vi "Individual Cartesian Measurements.vi"(6 "Forces In":dbl[](array[numeric]), 7 "LBCB Number":T1, 8 "error in (no error)":errorcluster, 9 "Displacements In":dbl[](array[numeric]), 11 "DAO Actions":T2) -> (0 "error out":errorcluster, 1 "Displacements Out":dbl[](array[numeric]), 5 "Forces Out":dbl[](array[numeric]))   [LabVIEW 2009]
uses:
  Data Access Objects/Metadata/DAO Actions.ctl
  Data Access Objects/Metadata/LBCB Number.ctl
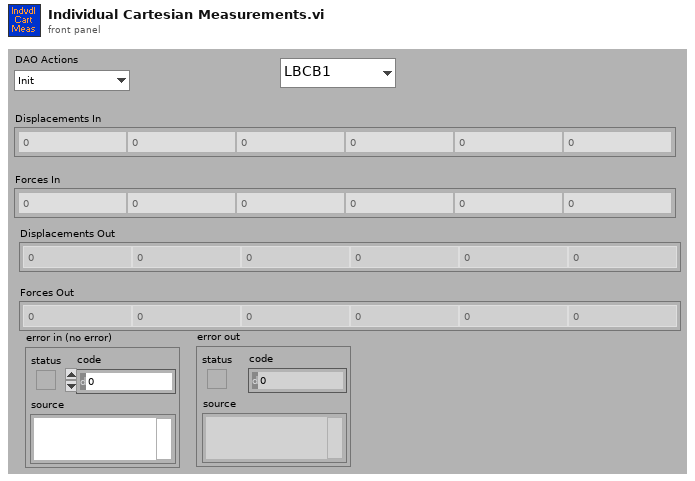
[diagram p1: front panel]
types:
  T1 = typedef "LBCB Number.ctl" = enum16{"LBCB1", "LBCB2"}
  T2 = typedef "DAO Actions.ctl" = enum16{"Init", "Get", "Set"}
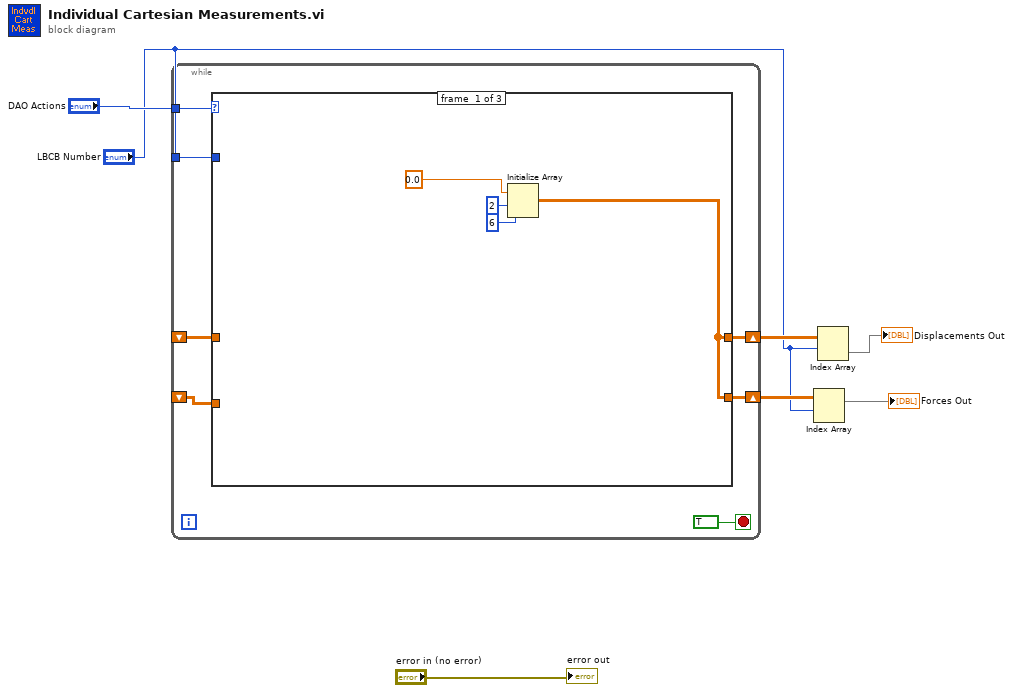
[diagram p0: block diagram]
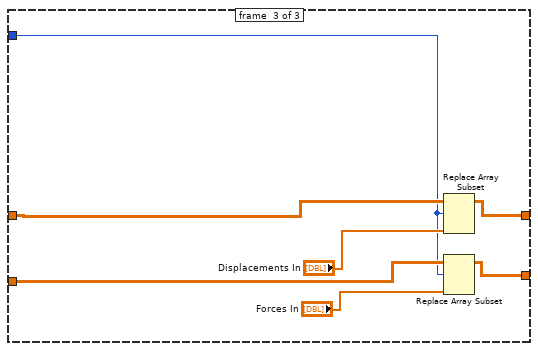
[diagram p3: hidden frame]
diagram:
  n1 = while {
    tunnel: "DAO Actions" -> [w13]
    shift-right: [w12] -> w5
    shift-left: _ -> [w11]
    tunnel: "LBCB Number" -> [w10]
    shift-right: [w9] -> w3
    shift-left: _ -> [w8]
    stop <- TRUE stop-if-true
    n2 = case shown="\"Get\"" w13 {
      tunnel: [w15 w20 w26] -> w12
      tunnel: w11 -> [_ w20 w27]
      tunnel: w10 -> [_ _ w21]
      tunnel: [w15 w19 w22] -> w9
      tunnel: w8 -> [_ w19 w23]
      frame #0 {
        n3 = Initialize Array(0.0, 2 ("dimension size"), 6 ("dimension size")) -> (w15:dbl[][])
      }
      frame #1 {
      }
      frame #2 {
        n4 = Replace Array Subset(array=w27, new element="Displacements In", index (row)=w21) -> (w26:dbl[][])  [unwired: 1 in]
        n5 = Replace Array Subset(array=w23, new element="Forces In", index (row)=w21) -> (w22:dbl[][])  [unwired: 1 in]
      }
    }
  }
  n6 = Index Array(array=w3, index (row)="LBCB Number") -> (element=→"Forces Out":dbl[])  [unwired: 1 in]
  n7 = Index Array(array=w5, index (row)="LBCB Number") -> (element=→"Displacements Out":dbl[])  [unwired: 1 in]
  "error out" <- "error in (no error)"
